vi "GCP_1k.vi"(8 "에러 출력":errorcluster, 10 "Period":sgl, 11 "Num":u32) -> (0 "에러 출력 2":errorcluster caption="에러 출력", 2 "GCP_1k":sgl)   [LabVIEW 2019]
uses:
  f716866b-1d7c-4ec3-a5f2-e1b712c7c0d6.vi
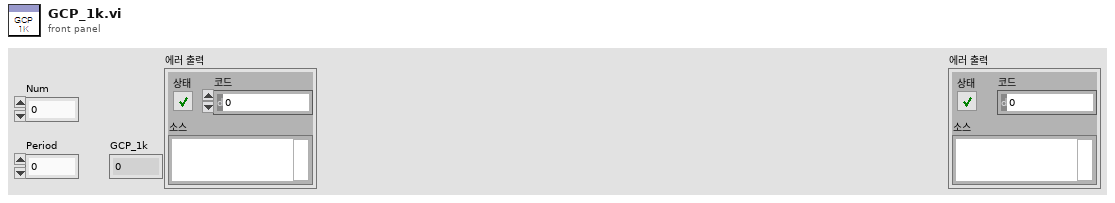
[diagram p1: front panel]
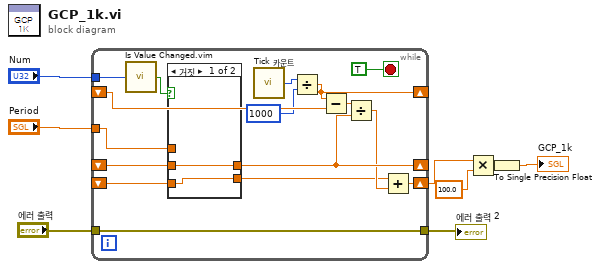
[diagram p0: block diagram]
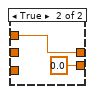
[diagram p2: hidden frame]
diagram:
  n1 = while {
    shift-right: [w22] -> _
    shift-left: _ -> [w23]
    shift-right: [w20] -> w4
    shift-left: _ -> [w19]
    shift-right: [w13] -> _
    shift-left: _ -> [w16]
    tunnel: "Period" -> [w12]
    tunnel: "Num" -> [w11]
    tunnel: "에러 출력" -> [w9]
    tunnel: [w9] -> w1
    stop <- TRUE stop-if-true
    n2 = call "Is Value Changed.vim"("value"=w11) -> ("changed or first call?"=w10:bool)
    n3 = case shown="거짓" w10 {
      tunnel: w12 -> [_ w28]
      tunnel: [w26 w28] -> w22
      tunnel: w23 -> [w26 _]
      tunnel: w19 -> [w25 _]
      tunnel: [w25 0.0] -> w18
      frame False {
      }
      frame True {
      }
    }
    n4 = call "Tick 카운트"() -> ("Tick Count(uSec)"=w15:u32)
    n5 = Divide(x=w15, y=u32 1000) -> (x/y=w13:dbl)
    n6 = Subtract(x=w13, y=w16) -> (x-y=w17:dbl)
    n7 = Divide(x=w17, y=w22) -> (x/y=w21:dbl)
    n8 = Add(x=w18, y=w21) -> (x+y=w20:dbl)
  }
  "에러 출력 2" <- w1
  n9 = Multiply(x=w4, y=100.0) -> (x*y=w3:dbl)
  n10 = To Single Precision Float(number=w3) -> (single precision float=→"GCP_1k":sgl)
